vi "Get Addresses for Setpoints.vi"(8 "error in (no error)":errorcluster, 10 "config file refnum in":T1, 11 "IED in":refnum<class "IED.lvclass">) -> (0 "error out":errorcluster, 2 "config file refnum out":T1, 3 "IED out":refnum<class "IED.lvclass">)   [LabVIEW 2015, in "IED Actor.lvlib" / "IED.lvclass"]
uses:
  IED.lvclass
  <vilib>/Utility/config.llb/Config Data RefNum.ctl
  <vilib>/NI/Tools/Keyed Array/KeyedArray.ctl
  IED.lvclass/IED.ctl
  <vilib>/NI/Tools/Keyed Array/Map String.vi
  <vilib>/NI/Tools/String/Get Case Matching.vi
  <vilib>/Utility/config.llb/Read Key (U32).vi
  <vilib>/Utility/config.llb/NI_LVConfig.lvlib
  <vilib>/NI/Tools/Keyed Array/Tools_KeyedArray.lvlib
  Utilities/Message Strings.llb/Message String Utilities.lvlib
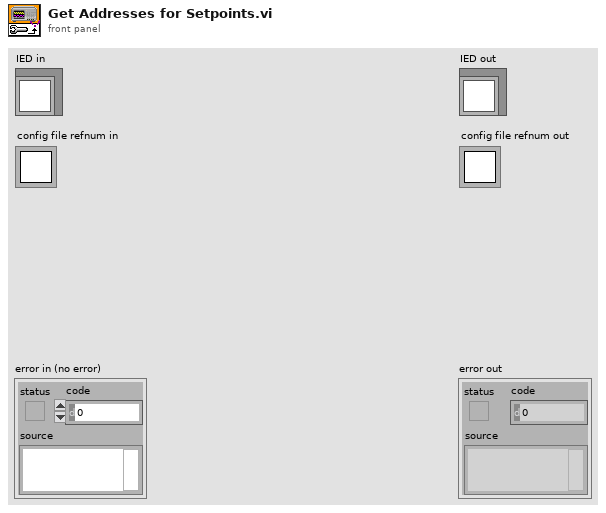
[diagram p1: front panel]
types:
  T1 = typedef "NI_LVConfig.lvlib/Config Data RefNum.ctl" = refnum<k1>
  T2 = typedef "Tools_KeyedArray.lvlib/KeyedArray.ctl" = cluster{"keys":string[], "values":string[]}
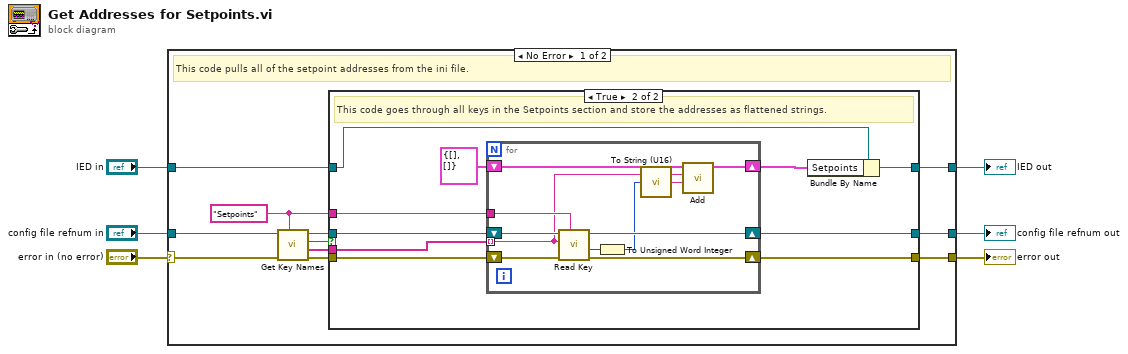
[diagram p0: block diagram]
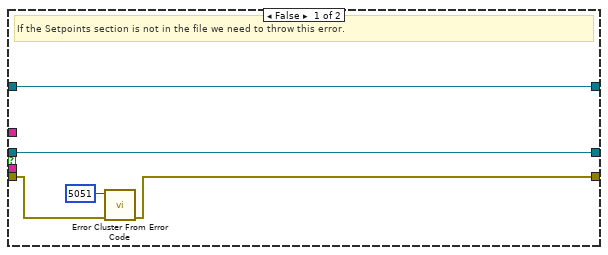
[diagram p2: hidden frame]
diagram:
  n1 = case shown="No Error" "error in (no error)" {
    selector: "error in (no error)" -> [w14 w46]
    tunnel: [w17 w46] -> w3
    tunnel: [w16 w45] -> w4
    tunnel: "IED in" -> [w7 w45]
    tunnel: "config file refnum in" -> [w15 w44]
    tunnel: [w9 w44] -> w1
    frame No Error {
      w8 = "Setpoints" ("section")
      # "This code pulls all of the setpoint addresses from the ini file."
      n2 = call <vilib>:"Get Key Names.vi"("section"=w8, "error in (no error)"=w14, "refnum"=w15) -> ("error out"=w10:errorcluster, "key names"=w11:string[], "section exists?"=w13:bool, "refnum out"=w12:T1)  [unwired: 5 in]
      n3 = case shown="True" w13 {
        tunnel: w7 -> [w19 w32]
        tunnel: [w20 w31] -> w17
        tunnel: [w19 w30] -> w16
        tunnel: w12 -> [w18 w27]
        tunnel: w11 -> [_ w28]
        tunnel: w10 -> [w22 w29]
        tunnel: [w18 w25] -> w9
        tunnel: w8 -> [_ w26]
        frame False {
          # "If the Setpoints section is not in the file we need to throw this error."
          n4 = call <vilib>:"Error Cluster From Error Code.vi"("error in (no error)"=w22, "error code (0)"=5051) -> ("error out"=w20:errorcluster)  [unwired: 7 in]
        }
        frame True {
          # "This code goes through all keys in the Setpoints section and store the addresses as flattened strings."
          n5 = for {
            shift-right: [w37] -> w31
            shift-left: w29 -> [w40]
            shift-right: [w42] -> w24
            shift-left: T2 {"keys"=[], "values"=[]} ("array out") -> [w43]
            tunnel: w28 -> [w33] mode=indexing
            tunnel: w26 -> [w39]
            shift-right: [w38] -> w25
            shift-left: w27 -> [w41]
            n6 = call-poly <vilib>:"Read Key.vi"("section"=w39, "error in (no error)"=w40, "key"=w33, "refnum"=w41) -> ("error out"=w37:errorcluster, "value"=w36:u32, "refnum out"=w38:T1)  [unwired: 4 in, 1 out]
            n7 = To Unsigned Word Integer(number=w36) -> (unsigned 16bit integer=w34:u16)
            n8 = call "To String (U16).vi"("UINT16 in"=w34) -> ("String out"=w35:string)
            n9 = call <vilib>:"Add.vi"("value"=w35, "key"=w33, "array in"=w43) -> ("array out"=w42:T2)  [unwired: 2 in, 2 out]
          }
          n10 = Bundle By Name(cluster=w32, "Setpoints"=w24) -> (w30:refnum<class "IED.lvclass">)
        }
      }
    }
    frame Error {
    }
  }
  "error out" <- w3
  "IED out" <- w4
  "config file refnum out" <- w1
